vi "Bold Row.vi"(8 "error in (no error)":errorcluster, 9 "Bold? (T)":bool=TRUE, 10 "Row (-2 : all)":i32=-2, 11 "MulticolumnListbox in":refnum<vi>) -> (0 "error out":errorcluster, 3 "MulticolumnListbox out":refnum<vi>)   [LabVIEW 2017, in "Engine Simulation Toolkit System Explorer.lvlib"]
uses:
  Engine Simulation Toolkit System Explorer.lvlib
  <vilib>/Utility/miscctls.llb/LVRowAndColumnTypeDef.ctl
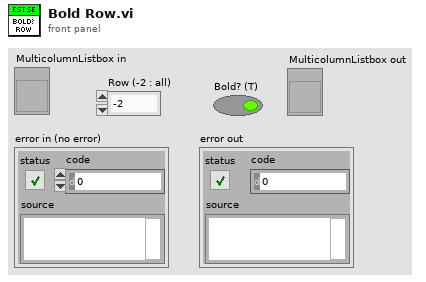
[diagram p1: front panel]
types:
  T1 = typedef "LVRowAndColumnTypeDef.ctl" = cluster{"Row":i32, "Column":i32}
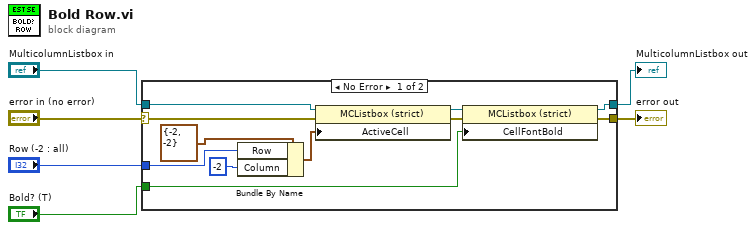
[diagram p0: block diagram]
diagram:
  n1 = case shown="No Error" "error in (no error)" {
    selector: "error in (no error)" -> [w17 w19]
    tunnel: "Bold? (T)" -> [w16 _]
    tunnel: "MulticolumnListbox in" -> [w14 w18]
    tunnel: "Row (-2 : all)" -> [w10 _]
    tunnel: [w9 w19] -> w2
    tunnel: [w8 w18] -> w1
    frame No Error {
      n2 = Bundle By Name(cluster=T1 {"Row"=-2, "Column"=-2} ("Active Cell:Active Cell"), "Row"=w10, "Column"=-2) -> (w12:T1)
      n3 = property on="Property Node" class="MCListbox (strict)"(reference=w14, error in=w17, "ActiveCell"=w12) -> (reference out=w7:refnum<vi>, error out=w15:errorcluster)
      n4 = property on="Property Node" class="MCListbox (strict)"(reference=w7, error in=w15, "CellFontBold"=w16) -> (reference out=w8:refnum<vi>, error out=w9:errorcluster)
    }
    frame Error {
    }
  }
  "error out" <- w2
  "MulticolumnListbox out" <- w1
